vi "GetFPMainPage.vi"(6 "错误输入（无错误）":errorcluster, 8 "索引":i32, 9 "Panel":refnum<vi>) -> (0 "错误输出":errorcluster, 3 "Page引用句柄":refnum<vi>)   [LabVIEW 2017]
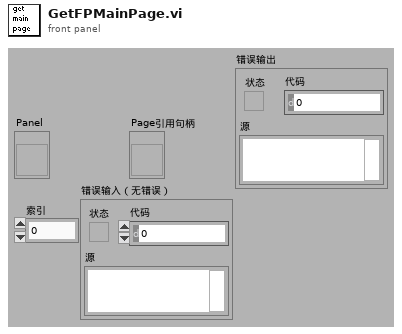
[diagram p1: front panel]
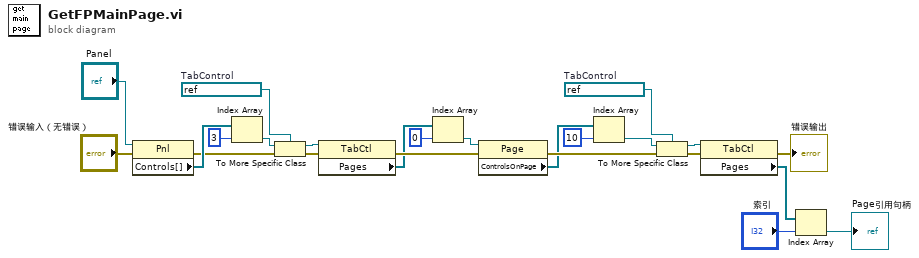
[diagram p0: block diagram]
diagram:
  w11 = refnum<vi> refnum  # TabControl
  w5 = refnum<vi> refnum  # TabControl
  n1 = property class="Pnl"(reference="Panel", error in="错误输入（无错误）") -> (error out=w9:errorcluster, "Controls[]"=w10:refnum<vi>[])  [unwired: 1 out]
  n2 = Index Array(array=w10, index=3 ("索引")) -> (element=w7:refnum<vi>)
  n3 = To More Specific Class(target class=w5, reference=w7, error in=w9) -> (specific class reference=w6:refnum<vi>, error out=w8:errorcluster)
  n4 = property class="TabCtl"(reference=w6, error in=w8) -> (error out=w18:errorcluster, "Pages"=w17:refnum<vi>[])  [unwired: 1 out]
  n5 = Index Array(array=w17, index=0 ("索引")) -> (element=w19:refnum<vi>)
  n6 = property class="Page"(reference=w19, error in=w18) -> (error out=w23:errorcluster, "ControlsOnPage"=w21:refnum<vi>[])  [unwired: 1 out]
  n7 = Index Array(array=w21, index=10 ("索引")) -> (element=w22:refnum<vi>)
  n8 = To More Specific Class(target class=w11, reference=w22, error in=w23) -> (specific class reference=w12:refnum<vi>, error out=w13:errorcluster)
  n9 = property class="TabCtl"(reference=w12, error in=w13) -> (error out=→"错误输出":errorcluster, "Pages"=w14:refnum<vi>[])  [unwired: 1 out]
  n10 = Index Array(array=w14, index="索引") -> (element=→"Page引用句柄":refnum<vi>)
